vi "Async.Engine.Initialize.vi"(5 "Custom Device Name":string, 6 "Timeout (ms) (5000)":u16=5000, 7 "Error Log Settings":T1, 8 "error in":errorcluster, 9 "Custom Device API in":refnum<class "Custom Device API.lvclass">, 10 "Processes":cluster{"VI":refnum<vi>, "Parameters":variant}[](array[cluster]), 11 "Compiled.InlineAsync.Settings":variant) -> (0 "error out":errorcluster, 3 "Async out":refnum<class "VS Inline Async API (Express).lvclass">)   [LabVIEW 2027, in "VS Inline Async API (Express).lvlib" / "VS Inline Async API (Express).lvclass"]
uses:
  VS Inline Async API (Express).lvclass
  Types/Error Handling Settings.ctl
  <userlib>/Custom Device Interfaces_v1.lvlibp/CustomDeviceAPI/Custom Device API.lvclass
  VS Inline Async API (Express).lvclass/VS Inline Async API (Express).ctl
  Error Handling Process/SubVIs/Error.GetError.vi
  Error Handling Process/Display and Log Process.vi
  <vilib>/Utility/error.llb/Error Cluster From Error Code.vi
  VS Inline Async API (Express).lvlib
  _Data Access Engine (Express)/Data Access Engine (Express)/Data Access Engine (Express).lvclass
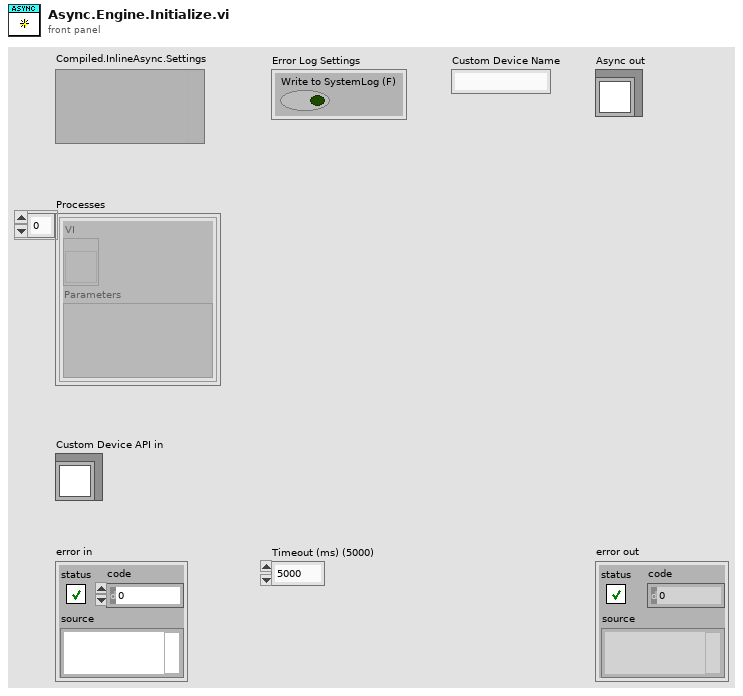
[diagram p1: front panel]
types:
  T1 = typedef "VS Inline Async API (Express).lvlib/VS Inline Async API (Express).lvclass/Error Handling Settings.ctl" = cluster{"Write to SystemLog (F)":bool}
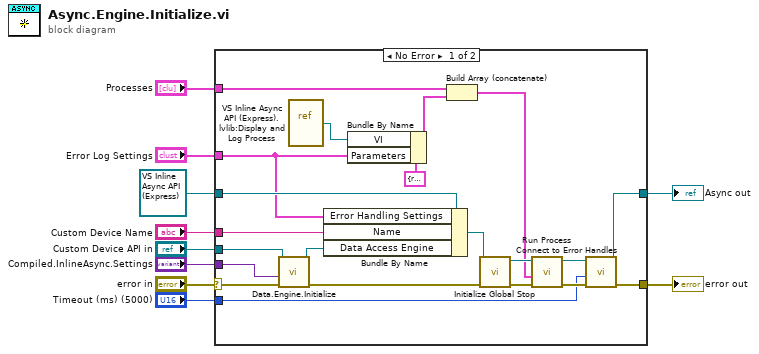
[diagram p0: block diagram]
diagram:
  n1 = case shown="No Error" "error in" {
    selector: "error in" -> [w19 w33]
    tunnel: [w28 w33] -> w9
    tunnel: [w26 w32] -> w1
    tunnel: refnum<class "VS Inline Async API (Express).lvclass"> refnum ("Async in") -> [w31 w32]
    tunnel: "Processes" -> [w30 _]
    tunnel: "Error Log Settings" -> [w17 _]
    tunnel: "Timeout (ms) (5000)" -> [w16 _]
    tunnel: "Custom Device API in" -> [w15 _]
    tunnel: "Compiled.InlineAsync.Settings" -> [w13 _]
    tunnel: "Custom Device Name" -> [w12 _]
    frame No Error {
      n2 = call "Data.Engine.Initialize.vi"("error in"=w19, "Compiled.InlineAsync.Settings"=w13, "Custom Device API in"=w15) -> ("error out"=w14:errorcluster, "Data Access Engine"=w11:refnum<class "Data Access Engine (Express).lvclass">)  [unwired: 7 in]
      n3 = vi-ref "VS Inline Async API (Express).lvlib:Display and Log Process.vi"() -> (w24:refnum<vi>)
      n4 = Bundle By Name(cluster=w31, "Error Handling Settings"=w17, "Name"=w12, "Data Access Engine"=w11) -> (w18:refnum<class "VS Inline Async API (Express).lvclass">)
      n5 = Bundle By Name(cluster=cluster{"VI":refnum<vi>, "Parameters":variant} {"VI"=refnum, "Parameters"=variant} ("Process"), "VI"=w24, "Parameters"=w17) -> (w23:cluster{"VI":refnum<vi>, "Parameters":variant})
      n6 = Build Array (concatenate)(w30, w23) -> (w20:cluster{"VI":refnum<vi>, "Parameters":variant}[])
      n7 = call "Initialize Global Stop.vi"("error in"=w14, "Async in"=w18) -> ("error out"=w22:errorcluster, "Async out"=w21:refnum<class "VS Inline Async API (Express).lvclass">)  [unwired: 8 in]
      n8 = call "Run Process.vi"("error in"=w22, "Processes"=w20, "Async in"=w21) -> ("error out"=w29:errorcluster, "Async out"=w27:refnum<class "VS Inline Async API (Express).lvclass">)  [unwired: 7 in]
      n9 = call "Connect to Error Handles.vi"("error in"=w29, "Timeout (ms)"=w16, "Async in"=w27) -> ("error out"=w28:errorcluster, "Async out"=w26:refnum<class "VS Inline Async API (Express).lvclass">)  [unwired: 7 in]
    }
    frame Error {
    }
  }
  "error out" <- w9
  "Async out" <- w1
